vi "Read.vi"(0 "reference in":refnum<class "DMM_Keysight_34980A.lvclass">, 5 "Samples":u32=1, 7 "dt":dbl, 9 "Timeout (10 s)":dbl=10000.0, 11 "error in (no error)":errorcluster) -> (4 "reference in":refnum<class "DMM_Keysight_34980A.lvclass">, 6 "Measurement":dbl[](array[numeric]), 8 "Time":dbl[](array[numeric]), 15 "error out":errorcluster)   [LabVIEW 2022 SP3, in "DMM_Keysight_34980A.lvlib" / "DMM_Keysight_34980A.lvclass"]
uses:
  DMM_Keysight_34980A.lvclass
  <vilib>/numeric/Random Number (Range) DBL.vi
  <vilib>/Waveform/WDTOps.llb/WDT Get Waveform Time Array DBL.vi
  <vilib>/measure/NI_MABase.lvlib
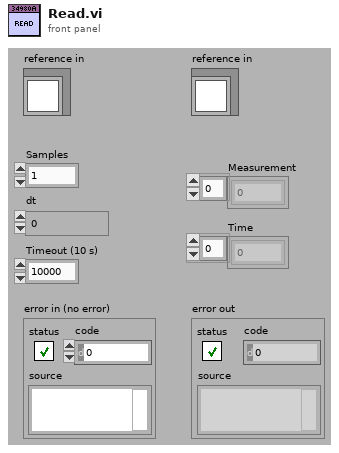
[diagram p1: front panel]
types:
  T1 = enum16{"Sine Wave", "Triangle Wave", "Square Wave", "Sawtooth Wave"}
  T2 = typedef "DMM_Keysight_34980A.lvlib/DMM_Keysight_34980A.lvclass/ObjectAttributes.ctl" = cluster{"Config":T3, "VISA ref":refnum<visa-resource-name>, "Meas":dbl, "Range DCV":enum16{"100 mV", "1 V", "10 V", "100 V", "300 V", "Auto", "Minimum", "Maximum"}, "Range ACV":enum16{"100 mV", "1 V", "10 V", "100 V", "300 V", "Auto", "Minimum", "Maximum", "Default"}, "Range Ohms":enum16{"100 Ohm", "1 kOhm", "10 kOhm", "100 kOhm", "1 MOhm", "10 MOhm", "100 MOhm", "Auto", "Minimum", "Maximum"}, "Range VFreq":enum16{"100 mV", "1 V", "10 V", "100 V", "300 V", "Auto", "Minimum", "Maximum"}, " Range ACA":enum16{"10 mA", "100 mA", "1 A", "Auto", "Minimum", "Maximum"}, " Range DCA":enum16{"10 mA", "100 mA", "1 A", "Auto", "Minimum", "Maximum"}, "Mode":T4, "Resolution":enum16{"4 1/2", "5 1/2", "6 1/2", "Least", "Highest", "Default"}, "Bandwidth":enum16{"3 Hz", "20 Hz", "200 Hz", "Minimum", "Maximum"}, "Low Frequency":enum16{"3 Hz", "20 Hz", "200 Hz", "Minimum", "Maximum"}, "Aperture":enum16{"10 ms", "100 ms", "1 sec", "Minimum", "Maximum"}, "Measurement":dbl[], "Time":dbl[], "Samples":u32, "dt":dbl, "Timeout":dbl}
  T3 = typedef "DMM_Keysight_34980A.lvlib/DMM_Keysight_34980A.lvclass/Config.ctl" = cluster{"VISA":refnum<visa-resource-name>}
  T4 = typedef "DMM_Keysight_34980A.lvlib/DMM_Keysight_34980A.lvclass/Mode.ctl" = enum16{"DCV", "ACV", "2W Ohms", "4W Ohms", "Frequency", "DCA", "ACA"}
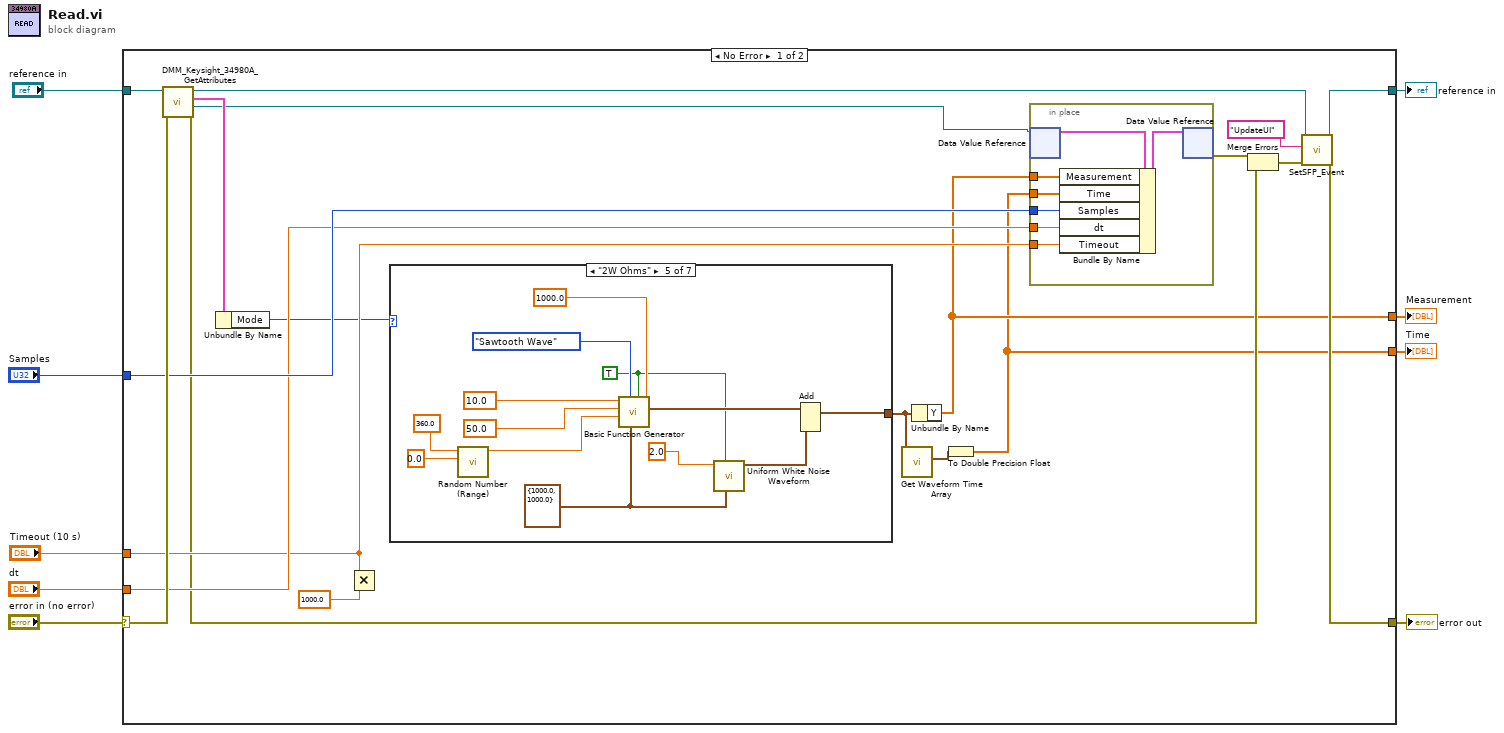
[diagram p0: block diagram]
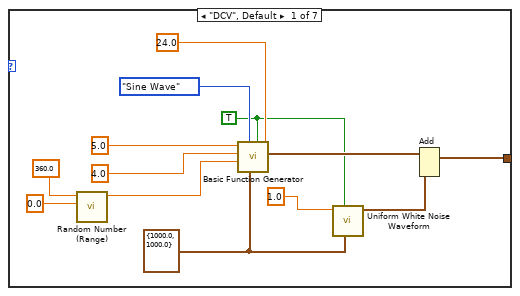
[diagram p2: hidden frame]
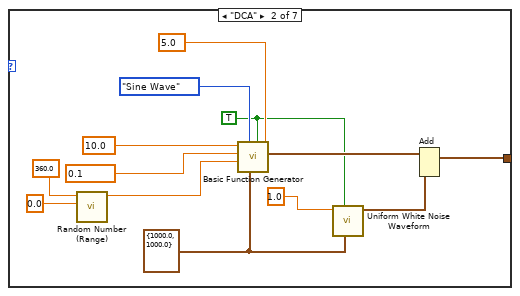
[diagram p3: hidden frame]
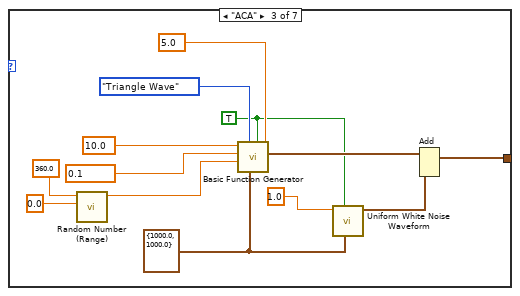
[diagram p4: hidden frame]
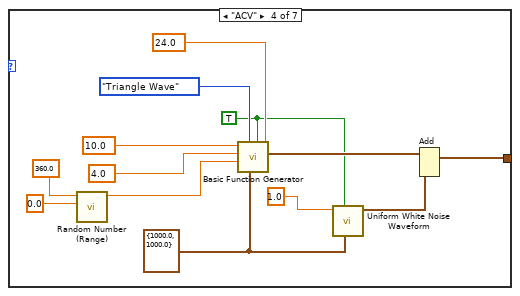
[diagram p5: hidden frame]
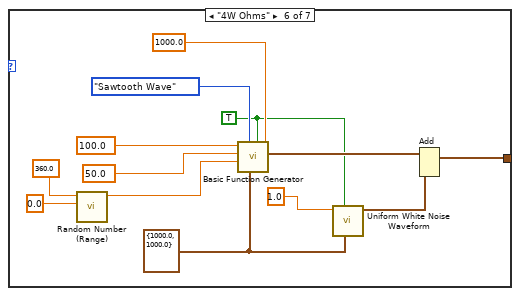
[diagram p6: hidden frame]
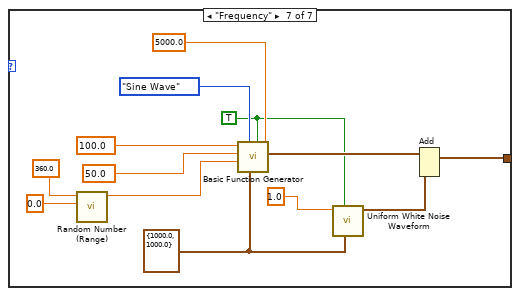
[diagram p7: hidden frame]
diagram:
  n1 = case shown="No Error" "error in (no error)" {
    selector: "error in (no error)" -> [w29 w129]
    tunnel: [w20 w129] -> w8
    tunnel: [w21 w128] -> w6
    tunnel: "reference in" -> [w27 w128]
    tunnel: "dt" -> [w18 _]
    tunnel: "Samples" -> [w19 _]
    tunnel: "Timeout (10 s)" -> [w16 _]
    tunnel: [w11 _] -> w2
    tunnel: [w10 _] -> w1
    frame No Error {
      n2 = call "DMM_Keysight_34980A_GetAttributes.vi"("error in (no error)"=w29, "reference in"=w27) -> ("error out"=w15:errorcluster, "DataRef"=w23:refnum<data-value>, "Data"=w28:T2, "reference out"=w22:refnum<class "DMM_Keysight_34980A.lvclass">)  [unwired: 6 in]
      n3 = Unbundle By Name(w28) -> ("Mode"=w14:T4)
      n4 = Multiply(x=w16, y=1000.0) -> ()  [unwired: 1 out]
      n5 = case shown="\"2W Ohms\"" w14 {
        tunnel: [w30 w43 w56 w69 w82 w95 w108] -> w13
        frame "DCV", Default {
          w37 = cluster{"Fs":dbl, "#s":dbl} {"Fs"=1000.0, "#s"=1000.0} ("sampling info")
          w34 = TRUE ("reset signal")
          n6 = call-poly <vilib>:"Random Number (Range).vi"("lower bound (0)"=0.0, "upper bound (100)"=360.0) -> ("number"=w31:dbl)  [unwired: 9 in]
          n7 = call <vilib>:"Basic Function Generator.vi"("offset"=24.0, "reset signal"=w34, "sampling info"=w37, "signal type"=T1."Sine Wave", "phase"=w31, "amplitude"=4.0 ("amplitude 2"), "frequency"=5.0) -> ("signal out"=w35:waveform(dbl))  [unwired: 2 in, 2 out]
          n8 = call <vilib>:"Uniform White Noise Waveform.vi"("sampling info"=w37, "reset signal"=w34, "amplitude"=1.0) -> ("signal out"=w36:waveform(dbl))  [unwired: 7 in, 1 out]
          n9 = Add(1:w36, 2:w35) -> (0:w30:waveform(dbl))  [unwired: 1 in, 1 out]
        }
        frame "DCA" {
          w50 = cluster{"Fs":dbl, "#s":dbl} {"Fs"=1000.0, "#s"=1000.0} ("sampling info")
          w47 = TRUE ("reset signal")
          n10 = call-poly <vilib>:"Random Number (Range).vi"("lower bound (0)"=0.0, "upper bound (100)"=360.0) -> ("number"=w44:dbl)  [unwired: 9 in]
          n11 = call <vilib>:"Basic Function Generator.vi"("offset"=5.0, "reset signal"=w47, "sampling info"=w50, "signal type"=T1."Sine Wave", "phase"=w44, "amplitude"=0.1 ("amplitude 2"), "frequency"=10.0) -> ("signal out"=w48:waveform(dbl))  [unwired: 2 in, 2 out]
          n12 = call <vilib>:"Uniform White Noise Waveform.vi"("sampling info"=w50, "reset signal"=w47, "amplitude"=1.0) -> ("signal out"=w49:waveform(dbl))  [unwired: 7 in, 1 out]
          n13 = Add(1:w49, 2:w48) -> (0:w43:waveform(dbl))  [unwired: 1 in, 1 out]
        }
        frame "ACA" {
          w63 = cluster{"Fs":dbl, "#s":dbl} {"Fs"=1000.0, "#s"=1000.0} ("sampling info")
          w60 = TRUE ("reset signal")
          n14 = call-poly <vilib>:"Random Number (Range).vi"("lower bound (0)"=0.0, "upper bound (100)"=360.0) -> ("number"=w57:dbl)  [unwired: 9 in]
          n15 = call <vilib>:"Basic Function Generator.vi"("offset"=5.0, "reset signal"=w60, "sampling info"=w63, "signal type"=T1."Triangle Wave", "phase"=w57, "amplitude"=0.1 ("amplitude 2"), "frequency"=10.0) -> ("signal out"=w61:waveform(dbl))  [unwired: 2 in, 2 out]
          n16 = call <vilib>:"Uniform White Noise Waveform.vi"("sampling info"=w63, "reset signal"=w60, "amplitude"=1.0) -> ("signal out"=w62:waveform(dbl))  [unwired: 7 in, 1 out]
          n17 = Add(1:w62, 2:w61) -> (0:w56:waveform(dbl))  [unwired: 1 in, 1 out]
        }
        frame "ACV" {
          w76 = cluster{"Fs":dbl, "#s":dbl} {"Fs"=1000.0, "#s"=1000.0} ("sampling info")
          w73 = TRUE ("reset signal")
          n18 = call-poly <vilib>:"Random Number (Range).vi"("lower bound (0)"=0.0, "upper bound (100)"=360.0) -> ("number"=w70:dbl)  [unwired: 9 in]
          n19 = call <vilib>:"Basic Function Generator.vi"("offset"=24.0, "reset signal"=w73, "sampling info"=w76, "signal type"=T1."Triangle Wave", "phase"=w70, "amplitude"=4.0 ("amplitude 2"), "frequency"=10.0) -> ("signal out"=w74:waveform(dbl))  [unwired: 2 in, 2 out]
          n20 = call <vilib>:"Uniform White Noise Waveform.vi"("sampling info"=w76, "reset signal"=w73, "amplitude"=1.0 ("amplitude 2")) -> ("signal out"=w75:waveform(dbl))  [unwired: 7 in, 1 out]
          n21 = Add(1:w75, 2:w74) -> (0:w69:waveform(dbl))  [unwired: 1 in, 1 out]
        }
        frame "2W Ohms" {
          w89 = cluster{"Fs":dbl, "#s":dbl} {"Fs"=1000.0, "#s"=1000.0} ("sampling info")
          w86 = TRUE ("reset signal")
          n22 = call-poly <vilib>:"Random Number (Range).vi"("lower bound (0)"=0.0, "upper bound (100)"=360.0) -> ("number"=w83:dbl)  [unwired: 9 in]
          n23 = call <vilib>:"Basic Function Generator.vi"("offset"=1000.0, "reset signal"=w86, "sampling info"=w89, "signal type"=T1."Sawtooth Wave", "phase"=w83, "amplitude"=50.0 ("amplitude 2"), "frequency"=10.0) -> ("signal out"=w87:waveform(dbl))  [unwired: 2 in, 2 out]
          n24 = call <vilib>:"Uniform White Noise Waveform.vi"("sampling info"=w89, "reset signal"=w86, "amplitude"=2.0 ("amplitude 2")) -> ("signal out"=w88:waveform(dbl))  [unwired: 7 in, 1 out]
          n25 = Add(1:w88, 2:w87) -> (0:w82:waveform(dbl))  [unwired: 1 in, 1 out]
        }
        frame "4W Ohms" {
          w102 = cluster{"Fs":dbl, "#s":dbl} {"Fs"=1000.0, "#s"=1000.0} ("sampling info")
          w99 = TRUE ("reset signal")
          n26 = call-poly <vilib>:"Random Number (Range).vi"("lower bound (0)"=0.0, "upper bound (100)"=360.0) -> ("number"=w96:dbl)  [unwired: 9 in]
          n27 = call <vilib>:"Basic Function Generator.vi"("offset"=1000.0, "reset signal"=w99, "sampling info"=w102, "signal type"=T1."Sawtooth Wave", "phase"=w96, "amplitude"=50.0 ("amplitude 2"), "frequency"=100.0) -> ("signal out"=w100:waveform(dbl))  [unwired: 2 in, 2 out]
          n28 = call <vilib>:"Uniform White Noise Waveform.vi"("sampling info"=w102, "reset signal"=w99, "amplitude"=1.0 ("amplitude 2")) -> ("signal out"=w101:waveform(dbl))  [unwired: 7 in, 1 out]
          n29 = Add(1:w101, 2:w100) -> (0:w95:waveform(dbl))  [unwired: 1 in, 1 out]
        }
        frame "Frequency" {
          w115 = cluster{"Fs":dbl, "#s":dbl} {"Fs"=1000.0, "#s"=1000.0} ("sampling info")
          w112 = TRUE ("reset signal")
          n30 = call-poly <vilib>:"Random Number (Range).vi"("lower bound (0)"=0.0, "upper bound (100)"=360.0) -> ("number"=w109:dbl)  [unwired: 9 in]
          n31 = call <vilib>:"Basic Function Generator.vi"("offset"=5000.0, "reset signal"=w112, "sampling info"=w115, "signal type"=T1."Sine Wave", "phase"=w109, "amplitude"=50.0 ("amplitude 2"), "frequency"=100.0) -> ("signal out"=w113:waveform(dbl))  [unwired: 2 in, 2 out]
          n32 = call <vilib>:"Uniform White Noise Waveform.vi"("sampling info"=w115, "reset signal"=w112, "amplitude"=1.0 ("amplitude 2")) -> ("signal out"=w114:waveform(dbl))  [unwired: 7 in, 1 out]
          n33 = Add(1:w114, 2:w113) -> (0:w108:waveform(dbl))  [unwired: 1 in, 1 out]
        }
      }
      n34 = call-poly <vilib>:"Get Waveform Time Array.vi"("waveform in"=w13) -> ("X array"=w12:timestamp[])  [unwired: 9 in, 1 out]
      n35 = Unbundle By Name(w13) -> ("Y"=w11:dbl[])
      n36 = To Double Precision Float(number=w12) -> (double precision float=w10:dbl[])
      n37 = in-place {
        in-place-border: w19 -> [w125]
        in-place-border: w18 -> [w124]
        in-place-border: w16 -> [w123]
        in-place-border: w11 -> [w122]
        in-place-border: w10 -> [w121]
        n38 = in-place-dvr #1(w23) -> (w127:T2)  [unwired: 1 out]
        n39 = Bundle By Name(cluster=w127, "Measurement"=w122, "Time"=w121, "Samples"=w125, "dt"=w124, "Timeout"=w123) -> (w126:T2)
        n40 = in-place-dvr #1(w126) -> (w26:errorcluster)  [unwired: 1 out]
      }
      n41 = Merge Errors(w26, w15) -> (w25:errorcluster)
      n42 = call-dynamic "SetSFP_Event.vi"("error in (no error)"=w25, "msg"="UpdateUI", "reference in"=w22) -> ("error out"=w20:errorcluster, "reference out"=w21:refnum<class "DMM_Keysight_34980A.lvclass">)  [unwired: 7 in]
    }
    frame Error {
    }
  }
  "error out" <- w8
  "reference in" <- w6
  "Measurement" <- w2
  "Time" <- w1
